vi "WildBugChilGru_V1.01.vi"() -> ()   [LabVIEW 2014]
uses:
  <vilib>/Utility/miscctls.llb/LVPointTypeDef.ctl
  <vilib>/Analysis/NI_AALBase.lvlib
  <vilib>/gmath/NI_Gmath.lvlib
  <vilib>/Analysis/NI_AALPro.lvlib
  <vilib>/Utility/xml.llb/Read From XML File(string).vi
  <vilib>/Utility/xml.llb/Write to XML File(string).vi
  <vilib>/Instr/_visa.llb/VISA Configure Serial Port (Instr).vi
  <vilib>/Analysis/3filter.llb/IIR Filter (DBL).vi
panel:
  in  "Registerkarte":T1(tab)
  in  "Zündung [Imp/U]":u8=1
  in  "Übersetzung ermitteln aus":T2(ring)
  in  "Getriebe [1:]":dbl=5.343
  in  "Reifenumfang [m]":dbl=1.222
  in  "Dauer [s]":dbl=5.0
  in  "nKuWe/nRolle":dbl=10.0
  in  "Lufttemperatur [°C]":dbl=20.0
  in  "Luftfeuchtigkeit [%]":dbl=50.0
  in  "Luftdruck [mbar]":dbl=1013.0
  in  "Messung Klimadaten":bool=TRUE
  in  "Gleitender Mittelwert":u8=35
  in  "Differenzenquotient":u8=12
  in  "Polynom":u8=15
  in  "n vom Gas [1/min]":dbl=5000.0
  in  "Rollengeber [Inkr/U]":u16=200
  in  "Rollenumfang [m]":dbl=0.613
  in  "Rollenträgheit [kgm²]":dbl=0.402
  in  "Recalc":bool
  in  "Ende":bool
  out "Datenspeicher":T3={"Fahrzeugdaten"="", "date/time string"="", "Rolle [Inkr/U]"=0, "Rollenumfang [m]"=0.0, "Rollenträgheit [kgm²]"=0.0, "Zündung [Imp/U]"=0, "Getriebe [1:]"=0.0, "Reifenumfang [m] "=0.0, "element"=0.0, "Gl. Mittelwert"=0, "Differenzenquotient"=0, "Polynom"=0, "element"=0.0, "element"=0.0, "Lufttemperatur [°C]"=0.0, "Luftfeuchtigkeit [%]"=0.0, "Luftdruck [mbar]"=0.0, [], [], "Best Polynomial Fit"=[], [], "Übersetzung ermitteln aus"=0, "[s]"=0.0, "nmin [1/min]"=0.0, "nmax [1/min]"=0.0, "n vom Gas [1/min]"=0.0, [], [], "Boolesch"=FALSE, "Serielle Schnittstelle"="COM4"}
  out "COM-Fehlerrate":string="0 / 0,0%"
  in  "Konfiguration:":bool
  in  "Speichern":bool
  in  "Drucken":bool
  out "Pmax":string="0,0 PS"
  out "Ergebnis":string="0,0 PS bei 0 1/min   |   0,0 Nm bei 0 1/min   |   vmax: 2147483647 km/h\nDIN 70020 k =1,000 (20 °C, 50 %, 1013 mbar)\n20.11.2016 20:05 "
  in  "Fahrzeugdaten":string="Hier die Fahrzeugdaten eingeben"
  out "XY-Graph":cluster{dbl[], dbl[]}[](graph)
  out "Untersetzung\nermittelt":bool
  out "Untersetzung":dbl format="%#.2f"
  in  "Start":bool
  out "Füllstand Lesepuffer":u64(slide) scale=1.0..100.0
  out "Hinterrad\n[km/h]":dbl(knob) scale=0.0..150.0
  out "Welle\n[1/min]":cluster{dbl, dbl}(knob) scale=0.0..12000.0
  out "Lesepuffer":string="\n"
  in  "Serielle Schnittstelle":refnum<visa-resource-name>="COM4"
  out "Untersetzung-Graph":dbl(graph)=2.6802446808510636 caption="Untersetzung"
  # "1. n konstant halten\n2. START\n3. n weiter halten\n4. bei GO: Vollgas\n5. vom Gas gehen"
  # "Zündung\nRolle"
  # "Untersetzung aus:"
  # "Eingabe <> Messen"
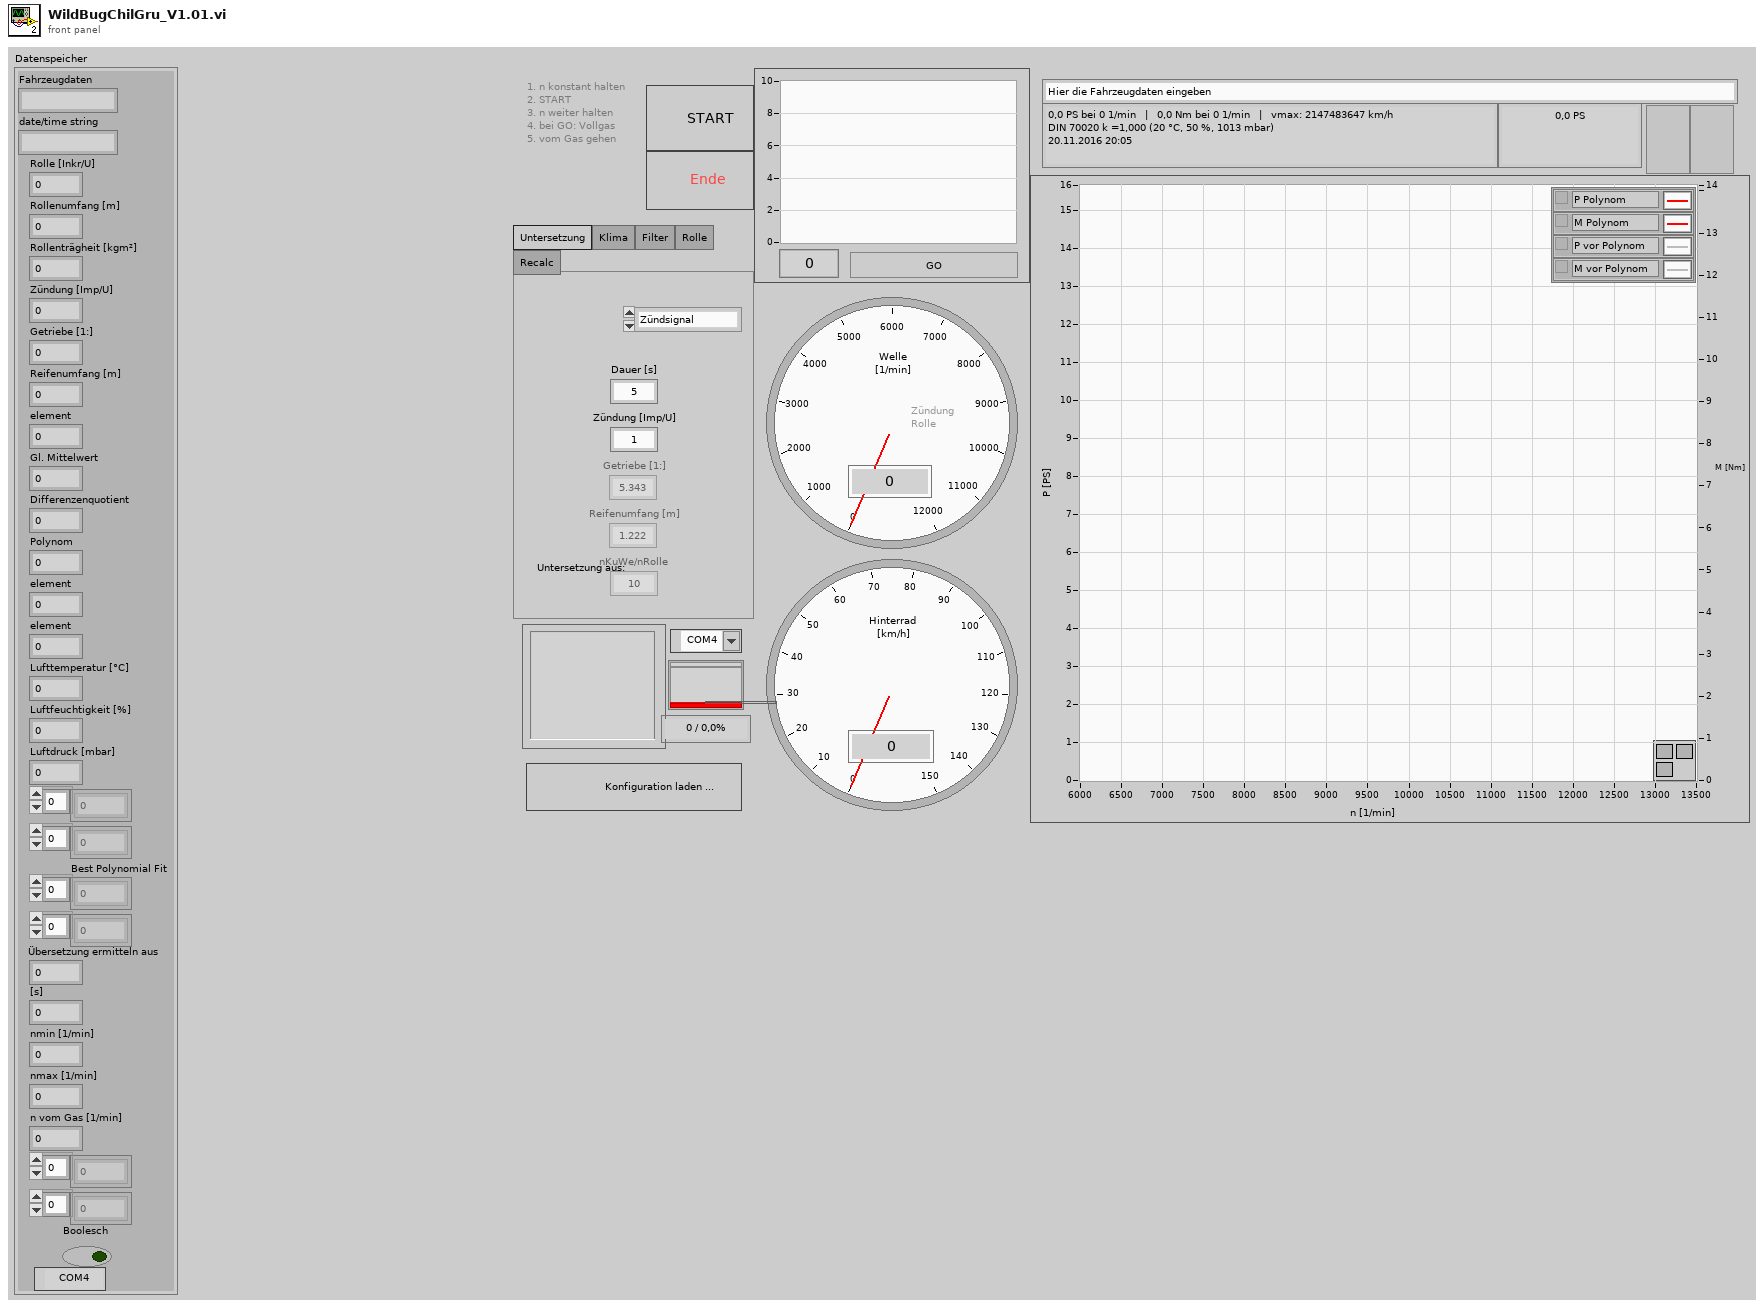
[diagram p1: front panel]
types:
  T1 = enum32{"Untersetzung", "Klima", "Filter", "Rolle", "Recalc"}
  T2 = enum8{"Zündsignal", "Getriebe & Reifen", "nKuWe / nRolle"}
  T3 = cluster{"Fahrzeugdaten":string, "date/time string":string, "Rolle [Inkr/U]":u16, "Rollenumfang [m]":dbl, "Rollenträgheit [kgm²]":dbl, "Zündung [Imp/U]":u8, "Getriebe [1:]":dbl, "Reifenumfang [m] ":dbl, "element":dbl, "Gl. Mittelwert":u8, "Differenzenquotient":u8, "Polynom":u8, "element":dbl, "element":dbl, "Lufttemperatur [°C]":dbl, "Luftfeuchtigkeit [%]":dbl, "Luftdruck [mbar]":dbl, dbl[], dbl[], "Best Polynomial Fit":dbl[], dbl[], "Übersetzung ermitteln aus":u8, "[s]":dbl, "nmin [1/min]":dbl, "nmax [1/min]":dbl, "n vom Gas [1/min]":dbl, dbl[], i32[], "Boolesch":bool, "Serielle Schnittstelle":refnum<visa-resource-name>}
  T4 = enum16{"Kleinste Quadrate", "Kleinestes absolutes Reiduum", "Biquadrat"}
  T5 = enum8{"Enabled", "Disabled", "Disabled and Grayed Out"}
  T6 = cluster{"Fahrzeugdaten":string, "date/time string":string, "Rollengeber [Inkr/U]":u16, "Rollenumfang [m]":dbl, "Rollenträgheit [kgm²]":dbl, "Zündung [Imp/U]":u8, "Getriebe [1:]":dbl, "Reifenumfang [m] ":dbl, "mean value":dbl, "Gleitender Mittelwert":u8, "Differenzenquotient":u8, "Polynom":u8, dbl, "element":dbl, "Lufttemperatur [°C]":dbl, "Luftfeuchtigkeit [%]":dbl, "Luftdruck [mbar]":dbl, dbl[], dbl[], "Best Polynomial Fit":dbl[], dbl[], "Übersetzung ermitteln aus":enum8{"Zündsignal", "Getriebe & Reifen", "nKuWe / nRolle"}, "Dauer [s]":dbl, dbl, dbl, "n vom Gas [1/min]":dbl, dbl[], i32[], "Messung Klimadaten":bool, "VISA resource name out":refnum<visa-resource-name>}
  T7 = typedef "LVPointTypeDef.ctl" = cluster{"Horizontal":i16, "Vertical":i16}
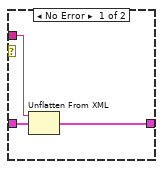
[diagram p2: hidden frame]
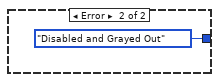
[diagram p3: hidden frame]
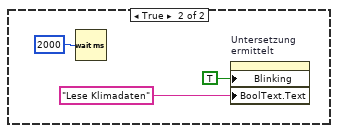
[diagram p5: hidden frame]
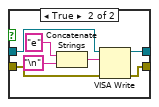
[diagram p6: hidden frame]
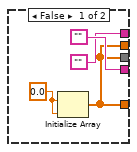
[diagram p8: hidden frame]
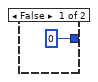
[diagram p9: hidden frame]
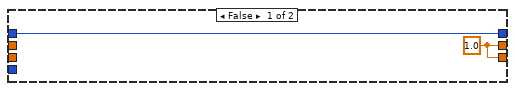
[diagram p11: hidden frame]
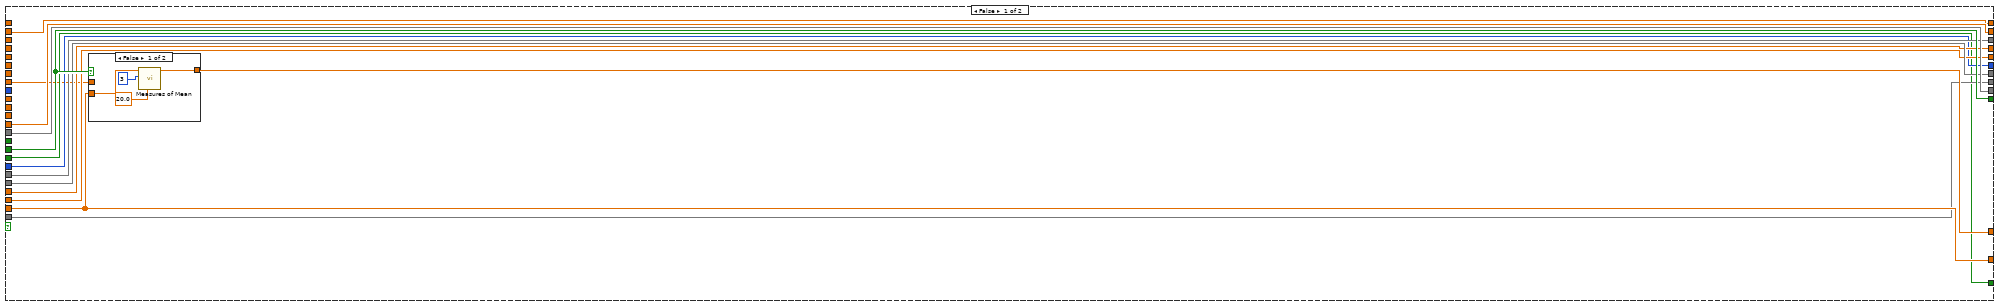
[diagram p12: hidden frame]
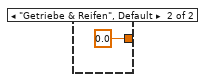
[diagram p16: hidden frame]
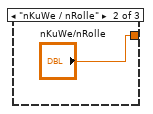
[diagram p18: hidden frame]
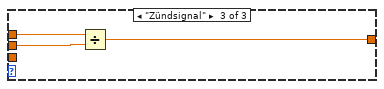
[diagram p19: hidden frame]
diagram:
  n1 = while {
    stop <- w1 stop-if-true
    n2 = event shown="[0] \"Start\": Wertänderung" {
      selector: _ -> [_ _]
      dyn-events: _ -> [_ _]
      timeout: _ -> [_ _]
      tunnel: [_ TRUE] -> w1
      event "Start": Value Change {
        n3 = event-data() -> ("NewVal"=w2:bool)  [unwired: 1 in, 5 out]
        n4 = case shown="True" w2 {
          frame False {
          }
          frame True {
            n5 = flat-sequence {
              tunnel: [w133] -> w118
              tunnel: [w132] -> w117
              tunnel: ["Messung Klimadaten"] -> w116
              tunnel: w118 -> [w146]
              tunnel: w117 -> [w145]
              tunnel: [0] -> w115
              tunnel: [1.0 ("element")] -> w114
              tunnel: [w143] -> w113
              tunnel: [w157] -> w112
              tunnel: [0] -> w111
              tunnel: [w143] -> w110
              tunnel: [-5] -> w109
              tunnel: [w154] -> w108
              tunnel: [w152] -> w107
              tunnel: [w151] -> w106
              tunnel: [0.0] -> w105
              tunnel: [w146] -> w104
              tunnel: [w145] -> w103
              tunnel: w116 -> [w144]
              tunnel: [w144] -> w102
              tunnel: w115 -> [w183]
              tunnel: [w183] -> w101
              tunnel: w114 -> [w182]
              tunnel: [w182] -> w100
              tunnel: w113 -> [w181]
              tunnel: [w181] -> w99
              tunnel: w112 -> [w180]
              tunnel: [w180] -> w98
              tunnel: w111 -> [w179]
              tunnel: [w179] -> w97
              tunnel: w110 -> [w178]
              tunnel: [w178] -> w96
              tunnel: w109 -> [w177]
              tunnel: [w177] -> w95
              tunnel: w108 -> [w176]
              tunnel: [w176] -> w94
              tunnel: w107 -> [w175]
              tunnel: [w175] -> w93
              tunnel: w106 -> [w174]
              tunnel: [w174] -> w92
              tunnel: w105 -> [w173]
              tunnel: [w173] -> w91
              tunnel: w104 -> [w172]
              tunnel: [w169] -> w90
              tunnel: w103 -> [w171]
              tunnel: [w170] -> w89
              tunnel: [w168] -> w88
              tunnel: w102 -> [w168]
              tunnel: w101 -> [w207]
              tunnel: [w207] -> w87
              tunnel: w100 -> [w206]
              tunnel: [w206] -> w86
              tunnel: w99 -> [w205]
              tunnel: [w205] -> w85
              tunnel: w98 -> [w204]
              tunnel: [w204] -> w84
              tunnel: w97 -> [w203]
              tunnel: [w203] -> w83
              tunnel: w96 -> [w202]
              tunnel: [w202] -> w82
              tunnel: w95 -> [w201]
              tunnel: [w201] -> w81
              tunnel: w94 -> [w200]
              tunnel: [w200] -> w80
              tunnel: w93 -> [w199]
              tunnel: [w199] -> w79
              tunnel: w92 -> [w198]
              tunnel: [w198] -> w78
              tunnel: w91 -> [w197]
              tunnel: [w197] -> w77
              tunnel: w90 -> [w196]
              tunnel: [w196] -> w76
              tunnel: w89 -> [w195]
              tunnel: [w195] -> w75
              tunnel: w88 -> [w193]
              tunnel: [w193] -> w74
              tunnel: w87 -> [w223]
              tunnel: [w223] -> w73
              tunnel: w86 -> [w222]
              tunnel: [w222] -> w72
              tunnel: w85 -> [w221]
              tunnel: [w221] -> w71
              tunnel: w84 -> [w220]
              tunnel: [w220] -> w70
              tunnel: w83 -> [w219]
              tunnel: [w219] -> w69
              tunnel: w82 -> [w218]
              tunnel: [w218] -> w68
              tunnel: w81 -> [w217]
              tunnel: [w217] -> w67
              tunnel: w80 -> [w216]
              tunnel: [w216] -> w66
              tunnel: w79 -> [w215]
              tunnel: [w215] -> w65
              tunnel: w78 -> [w214]
              tunnel: [w214] -> w64
              tunnel: w77 -> [w213]
              tunnel: [w213] -> w63
              tunnel: w76 -> [w212]
              tunnel: [w211] -> w62
              tunnel: w75 -> [w209]
              tunnel: [w210] -> w61
              tunnel: w74 -> [w208]
              tunnel: w73 -> [w297]
              tunnel: w72 -> [w296]
              tunnel: w71 -> [w295]
              tunnel: w70 -> [w294]
              tunnel: w69 -> [w293]
              tunnel: w68 -> [w292]
              tunnel: w67 -> [w291]
              tunnel: w66 -> [w290]
              tunnel: w65 -> [w289]
              tunnel: w64 -> [w288]
              tunnel: w63 -> [w287]
              tunnel: w62 -> [w252]
              tunnel: [w297] -> w60
              tunnel: [w296] -> w59
              tunnel: [w295] -> w58
              tunnel: [w294] -> w57
              tunnel: [w293] -> w56
              tunnel: [w292] -> w55
              tunnel: [w291] -> w54
              tunnel: [w290] -> w53
              tunnel: [w289] -> w52
              tunnel: [w288] -> w51
              tunnel: [w287] -> w50
              tunnel: [w252] -> w49
              tunnel: [w251] -> w48
              tunnel: [w286] -> w47
              tunnel: [w285] -> w46
              tunnel: [w284] -> w45
              tunnel: ["Gleitender Mittelwert"] -> w44
              tunnel: w61 -> [w251]
              tunnel: [w306] -> w10
              tunnel: [w307] -> w11
              tunnel: [w308] -> w12
              tunnel: [w309] -> w13
              tunnel: [w300] -> w8
              tunnel: [w299] -> w9
              tunnel: [w310] -> w14
              tunnel: [w311] -> w15
              tunnel: [w312] -> w17
              tunnel: [w313] -> w19
              tunnel: [w314] -> w20
              tunnel: [w315] -> w21
              tunnel: [w316] -> w38
              tunnel: [w317] -> w40
              tunnel: [w318] -> w41
              tunnel: [w319] -> w42
              tunnel: [w320] -> w43
              tunnel: w60 -> [w320]
              tunnel: w59 -> [w319]
              tunnel: w58 -> [w318]
              tunnel: w57 -> [w317]
              tunnel: w56 -> [w316]
              tunnel: w55 -> [w315]
              tunnel: w54 -> [w314]
              tunnel: w53 -> [w313]
              tunnel: w52 -> [w312]
              tunnel: w51 -> [w311]
              tunnel: w50 -> [w310]
              tunnel: w49 -> [w302]
              tunnel: w48 -> [w301]
              tunnel: w47 -> [w309]
              tunnel: w46 -> [w308]
              tunnel: w45 -> [w307]
              tunnel: w44 -> [w306]
              frame #0 {
                w138 = u16 0 items=["None", "XON/XOFF", "RTS/CTS", "XON/XOFF & RTS/CTS", "DTR/DSR", "XON/XOFF & DTR/DSR"] ("flow control (0:none)")
                w139 = u16 10 items=["1.0"=10, "1.5"=15, "2.0"=20] ("stop bits (10: 1 bit)")
                w131 = FALSE  # Enable Termination Char (T)
                w134 = u32 10000  # timeout (10sec)
                n6 = call-poly "VISA Configure Serial Port"("VISA resource name"="Serielle Schnittstelle", "timeout (10sec)"=w134, "Enable Termination\nChar (T)"=w131, "baud rate (9600)"=u32 115200 ("baudrate (250000)"), "data bits (8)"=u16 8, "parity (0:none)"=enum16{"None", "Odd", "Even", "Mark", "Space"}."None", "stop bits (10: 1 bit)"=w139, "flow control (0:none)"=w138) -> ("VISA resource name out"=w136:refnum<visa-resource-name>, "error out"=w135:errorcluster)  [unwired: 6 in]
                n7 = VISA Clear(VISA resource name=w136, error in (no error)=w135) -> (VISA resource name out=w133:refnum<visa-resource-name>, error out=w132:errorcluster)
              }
              frame #1 {
                w147 = T5."Disabled and Grayed Out" ("Deaktiviert")
                w150 = 0.0  # Graphen löschen
                w153 = 0
                w158 = 0.0
                w143 = FALSE
                w151 = ""
                n8 = case shown="False" w144 {
                  frame False {
                    n9 = property on="Untersetzung\nermittelt" class="Bool. (strikt)"("Blinking"=TRUE ("Blinkend"), "BoolText.Text"="Initialisiere" ("Beschriftung.Text")) -> ()  [unwired: 2 in, 2 out]
                  }
                  frame True {
                    n10 = Wait (ms)(milliseconds to wait=u32 2000 ("Zu wartende ms")) -> ()  [unwired: 1 out]
                    n11 = property on="Untersetzung\nermittelt" class="Bool. (strikt)"("Blinking"=TRUE ("Blinkend"), "BoolText.Text"="Lese Klimadaten" ("Beschriftung.Text")) -> ()  [unwired: 2 in, 2 out]
                  }
                }
                n12 = Build Array(w150) -> (w149:dbl[])
                n13 = property on="Untersetzung-Graph" class="SVDiagr (strikt)"("History Data"=w149) -> ()  [unwired: 2 in, 2 out]
                n14 = property on="Drucken" class="Bool. (strikt)"("DisabledEnum"=w147) -> ()  [unwired: 2 in, 2 out]
                n15 = property on="Übersetzung ermitteln aus" class="Enum (strikt)"("DisabledEnum"=w147) -> ()  [unwired: 2 in, 2 out]
                n16 = property on="Konfiguration:" class="Bool. (strikt)"("DisabledEnum"=w147) -> ()  [unwired: 2 in, 2 out]
                n17 = property on="Ende" class="Bool. (strikt)"("DisabledEnum"=w147) -> ()  [unwired: 2 in, 2 out]
                n18 = property on="Speichern" class="Bool. (strikt)"("DisabledEnum"=w147) -> ()  [unwired: 2 in, 2 out]
                n19 = local write "Pmax"(w151) -> ()
                n20 = local write "COM-Fehlerrate"(w151) -> ()
                n21 = local write "Ergebnis"(w151) -> ()
                n22 = Initialize Array(w158, w158) -> (w157:dbl[])
                n23 = Initialize Array(0.0 ("y"), 0) -> (w154:dbl[])
                n24 = Initialize Array(w153, w153) -> (w152:i32[])
              }
              frame #2 {
                n25 = case shown="False" w168 {
                  tunnel: w172 -> [w185 w189]
                  tunnel: w171 -> [w184 w188]
                  tunnel: [w184 w187] -> w170
                  tunnel: [w185 w186] -> w169
                  frame False {
                  }
                  frame True {
                    n26 = Concatenate Strings("e" ("String"), "\n") -> (w192:string)
                    n27 = VISA Write(VISA resource name=w189, write buffer=w192, error in (no error)=w188) -> (VISA resource name out=w186:refnum<visa-resource-name>, error out=w187:errorcluster)  [unwired: 1 out]
                  }
                }
              }
              frame #3 {
                n28 = Wait (ms)(milliseconds to wait=u32 500 ("Zu wartende ms")) -> ()  [unwired: 1 out]
              }
              frame #4 {
                n29 = case shown="True" w208 {
                  tunnel: w212 -> [w225 w246]
                  tunnel: [w225 w245] -> w211
                  tunnel: [w224 w244] -> w210
                  tunnel: w209 -> [w224 w243]
                  frame False {
                  }
                  frame True {
                    w228 = ";" ("Regulärer Ausdruck")
                    n30 = property class="Instr"(reference=w246, error in=w243) -> (reference out=w249:refnum<visa-resource-name>, error out=w248:errorcluster, "Serial Settings:Number of Bytes at Serial Port"=w247:u32)
                    n31 = VISA Read(VISA resource name=w249, byte count=w247, error in (no error)=w248) -> (VISA resource name out=w245:refnum<visa-resource-name>, read buffer=w240:string, error out=w244:errorcluster)  [unwired: 1 out]
                    n32 = Search and Replace String(replace all?=TRUE ("Alle ersetzen? (F)"), input string=w240, search string="." ("Such-String"), replace string="," ("Ersetzungs-String (\"\")")) -> (result string=w233:string)  [unwired: 4 in, 3 out]
                    n33 = Match Pattern(string=w233, regular expression=w228) -> (before substring=w231:string, after substring=w232:string)  [unwired: 1 in, 2 out]
                    n34 = Match Pattern(string=w232, regular expression=w228) -> (before substring=w230:string, after substring=w229:string)  [unwired: 1 in, 2 out]
                    n35 = Fract/Exp String To Number(string=w231, offset=0 ("Offset")) -> (number=w239:dbl)  [unwired: 2 in, 1 out]
                    n36 = local write "Lufttemperatur [°C]"(w239) -> ()
                    n37 = Fract/Exp String To Number(string=w230) -> (number=w236:dbl)  [unwired: 3 in, 1 out]
                    n38 = Match Pattern(string=w229, regular expression=w228) -> (before substring=w227:string)  [unwired: 1 in, 3 out]
                    n39 = Fract/Exp String To Number(string=w227) -> (number=w238:dbl)  [unwired: 3 in, 1 out]
                    n40 = Divide(x=w236, y=100.0 ("x")) -> (x/y=w237:dbl)
                    n41 = local write "Luftdruck [mbar]"(w237) -> ()
                    n42 = local write "Luftfeuchtigkeit [%]"(w238) -> ()
                  }
                }
              }
              frame #5 {
                n43 = Wait (ms)(milliseconds to wait=u32 2000 ("Zu wartende ms")) -> ()  [unwired: 1 out]
                n44 = Add(x="Lufttemperatur [°C]", y=273.15) -> (x+y=w267:dbl)
                n45 = Divide ("M_Welle [Nm]")(x=300.0, y=w267) -> (x/y=w270:dbl)
                n46 = Multiply(x="Luftfeuchtigkeit [%]", y=0.01) -> (x*y=w281:dbl)
                n47 = Divide ("M_Welle [Nm]")(x=w267, y=293.15) -> (x/y=w265:dbl)
                n48 = Multiply(x=w281, y=240800000000.0) -> (x*y=w255:dbl)
                n49 = Power Of X(1:w270, 2:5.0) -> (0:w268:dbl)
                n50 = Multiply(x=w255, y=w268) -> (x*y=w275:dbl)
                n51 = Multiply(x=w270, y=-22.644) -> (x*y=w276:dbl)
                n52 = Power Of X(1:w265, 2:0.5) -> (0:w262:dbl)
                n53 = Exponential(1:w276) -> (0:w274:dbl)
                n54 = Multiply(x=w275, y=w274) -> (x*y=w273:dbl)
                n55 = Subtract "p_Trocken [mbar]"(x="Luftdruck [mbar]", y=w273) -> (x-y=w271:dbl)
                n56 = Divide ("M_Welle [Nm]")(x=1013.0, y=w271) -> (x/y=w263:dbl)
                n57 = Multiply "Korrekturfaktor DIN 70020"(x=w263, y=w262) -> (x*y=w286:dbl)
                n58 = Divide(x="Gleitender Mittelwert", y=2) -> (x/y=w259:dbl)
                n59 = Round Toward -Infinity(1:w259) -> (0:w258:dbl)
                n60 = call <vilib>:"Smoothing Filter Coefficients.vi"("shape"=1, "half-width"=w258, "type"=0) -> ("forward coefficients"=w284:dbl[], "reverse coefficients"=w285:dbl[])  [unwired: 6 in, 1 out]
              }
              frame #6 {
                n61 = Concatenate Strings("m" ("String"), "\n") -> (w305:string)
                n62 = property on="Untersetzung\nermittelt" class="Bool. (strikt)"("Blinking"=FALSE ("Blinkend")) -> ()  [unwired: 2 in, 2 out]
                n63 = VISA Write(VISA resource name=w302, write buffer=w305, error in (no error)=w301) -> (VISA resource name out=w299:refnum<visa-resource-name>, error out=w300:errorcluster)  [unwired: 1 out]
              }
            }
            n64 = while {
              tunnel: w9 -> [w453]
              tunnel: w8 -> [w452]
              shift-right: [w523] -> _
              shift-left: w15 -> [w468]
              shift-right: [w518] -> _
              shift-left: w14 -> [w522]
              shift-right: [w517] -> _
              shift-left: w14 -> [w521]
              shift-right: [w472] -> _
              shift-left: w14 -> [w520]
              shift-right: [w499] -> _
              shift-left: w43 -> [w519]
              shift-right: [w460] -> w26
              shift-left: w42 -> [_]
              shift-right: [w478] -> w30
              shift-left: w14 -> [w500]
              shift-right: [w510] -> w28
              shift-left: w14 -> [w474]
              shift-right: [w473] -> _
              shift-left: w19 -> [w514]
              shift-right: [w511] -> _
              shift-left: w41 -> [w488]
              shift-right: [w454] -> _
              shift-left: w40 -> [_]
              shift-right: [w459] -> _
              shift-left: w40 -> [_]
              shift-right: [w509] -> w29
              shift-left: w40 -> [w507]
              shift-right: [w508] -> _
              shift-left: w40 -> [w506]
              shift-right: [w494] -> w37
              shift-left: w19 -> [w505]
              shift-right: [w498] -> _
              shift-left: w19 -> [w503]
              shift-right: [w497] -> w33
              shift-left: w19 -> [w504]
              shift-right: [w496] -> w36
              shift-left: w19 -> [w502]
              shift-right: [w495] -> w35
              shift-left: w19 -> [w501]
              tunnel: [w493] -> w39
              shift-right: [w489] -> w34
              shift-left: w38 -> [w491]
              tunnel: [w492] -> w5
              tunnel: ["n vom Gas [1/min]"] -> w32
              tunnel: ["Rollenumfang [m]"] -> w31
              tunnel: ["Rollenumfang [m]"] -> w25
              shift-right: [w485] -> _
              shift-left: w21 -> [w451]
              shift-right: [w479] -> _
              shift-left: w20 -> [w484]
              shift-right: [w480] -> _
              shift-left: w14 -> [w483]
              shift-right: [w481] -> _
              shift-left: w14 -> [w482]
              shift-right: [w477] -> w18
              shift-left: w19 -> [w476]
              shift-right: [w471] -> _
              shift-left: _ -> [w470]
              shift-right: [w475] -> w16
              shift-left: w17 -> [w469]
              tunnel: [w467] -> w6
              tunnel: w13 -> [w460]
              tunnel: w12 -> [w454]
              tunnel: w11 -> [w459]
              tunnel: w10 -> [w458]
              stop <- w493 stop-if-true
              n65 = property class="Instr"(reference=w453, error in=w452) -> (reference out=w463:refnum<visa-resource-name>, error out=w462:errorcluster, "Serial Settings:Number of Bytes at Serial Port"=w465:u32)
              n66 = Greater?(x=w465, y=u32 1 ("min. Bytes")) -> (0:w461:bool)
              n67 = case shown="True" w461 {
                tunnel: w465 -> [_ w525]
                tunnel: [u32 0 ("Bytes at Port") w525] -> w464
                frame False {
                }
                frame True {
                }
              }
              n68 = case shown="1.." w464 {
                selector: w464 -> [_ w778]
                tunnel: [w728 w772] -> w492
                tunnel: [w727 w773] -> w467
                tunnel: [w732 w774] -> w517
                tunnel: [w733 w771] -> w518
                tunnel: w468 -> [w734 w769]
                tunnel: [w734 w767] -> w523
                tunnel: w522 -> [w733 w759]
                tunnel: w521 -> [w732 w758]
                tunnel: [w729 w757] -> w472
                tunnel: w520 -> [w729 w756]
                tunnel: w519 -> [w731 _]
                tunnel: [w731 w739] -> w499
                tunnel: [w730 w745] -> w471
                tunnel: w470 -> [w730 w744]
                tunnel: w463 -> [w727 w736]
                tunnel: w462 -> [w728 w735]
                frame 0, Default {
                  # "No data in from serial port - Nothing to do."
                }
                frame 1.. {
                  # "Hz Drum"
                  n69 = VISA Read(VISA resource name=w736, byte count=w778, error in (no error)=w735) -> (VISA resource name out=w773:refnum<visa-resource-name>, read buffer=w770:string, error out=w772:errorcluster)  [unwired: 1 out]
                  n70 = Concatenate Strings(w769, w770) -> (w741:string)
                  "Lesepuffer" <- w741
                  n71 = Spreadsheet String To Array(delimiter (Tab)="\n" ("regular expression"), format string="%s" ("regular expression"), spreadsheet string=w741, array type (2D Dbl)=string[] [] ("Array 2")) -> (array=w750:string[])
                  n72 = Match Pattern(string=w741, regular expression="[\\n]") -> (before substring=w748:string, after substring=w768:string, offset past match=w782:i32)  [unwired: 1 in, 1 out]
                  n73 = Array Size(array=w750) -> (size(s)=w754:i32)
                  n74 = Match Pattern(string=w748, regular expression="[;]") -> (before substring=w746:string, after substring=w747:string, offset past match=w743:i32)  [unwired: 1 in, 1 out]
                  n75 = Subtract "aktuelle Zeilenanzahl"(x=w754, y=1) -> (x-y=w739:i32)
                  n76 = property on="Füllstand Lesepuffer" class="Schieber (strikt)"() -> ("Scale.Maximum"=w738:dbl)  [unwired: 2 in, 2 out]
                  n77 = Match Pattern(string=w747, regular expression="[;]") -> (before substring=w777:string, after substring=w780:string, offset past match=w765:i32)  [unwired: 1 in, 1 out]
                  n78 = Match Pattern(string=w780, regular expression="[;]") -> (before substring=w776:string, after substring=w775:string, offset past match=w763:i32)  [unwired: 1 in, 1 out]
                  n79 = Greater Or Equal To 0?(x=w743) -> (x >= 0?=w742:bool)
                  n80 = Greater?(x=w739, y=w738) -> (0:w740:bool)
                  n81 = Greater Or Equal To 0?(x=w763) -> (x >= 0?=w762:bool)
                  n82 = Greater Or Equal To 0?(x=w765) -> (x >= 0?=w764:bool)
                  n83 = Greater Or Equal To 0?(x=w782) -> (x >= 0?=w766:bool)
                  n84 = Select(t=w739, s=w740, f=w738) -> (s? t:f=w737:dbl)
                  n85 = Build Array(w766, w764, w742, w762) -> (w761:bool[])
                  n86 = property on="Füllstand Lesepuffer" class="Schieber (strikt)"("Scale.Maximum"=w737) -> ()  [unwired: 2 in, 2 out]
                  n87 = And Array Elements(Boolean array=w761) -> (logical AND=w760:bool)
                  n88 = case shown="True" w760 {
                    tunnel: w777 -> [_ w793]
                    tunnel: w776 -> [_ w798]
                    tunnel: w775 -> [_ w797]
                    tunnel: [w786 w796] -> w774
                    tunnel: [w787 w795] -> w771
                    tunnel: w768 -> [_ w794]
                    tunnel: [w788 w794] -> w767
                    tunnel: w741 -> [w788 _]
                    tunnel: w759 -> [w787 _]
                    tunnel: w758 -> [w786 _]
                    tunnel: [w785 w792] -> w757
                    tunnel: w756 -> [w785 _]
                    tunnel: w746 -> [_ w791]
                    tunnel: [w784 w789] -> w745
                    tunnel: w744 -> [w784 _]
                    frame False {
                    }
                    frame True {
                      # "Cyclecounter"
                      # "Hz ComLevel"
                      # "ComLevel\nLevel 10 =   6Hz \nLevel 5 =   12Hz \nLevel 4 =   15Hz\nLevel 3 =   20Hz\nLevel 2 =   33Hz\nLevel 1 =   62Hz"
                      # "Hz Drum"
                      # "Hz Engine"
                      # "t4m"
                      n89 = Fract/Exp String To Number(string=w791) -> (number=w790:dbl)  [unwired: 3 in, 1 out]
                      n90 = Fract/Exp String To Number(string=w797) -> (number=w796:dbl)  [unwired: 3 in, 1 out]
                      n91 = Fract/Exp String To Number(string=w793) -> (number=w792:dbl)  [unwired: 3 in, 1 out]
                      n92 = To Long Integer(number=w790) -> (32bit integer=w789:i32)
                      n93 = Fract/Exp String To Number(string=w798) -> (number=w795:dbl)  [unwired: 3 in, 1 out]
                    }
                  }
                }
              }
              "Füllstand Lesepuffer" <- w499
              n94 = Not Equal?(x=w470, y=w471) -> (x != y?=w455:bool)
              n95 = case shown="True" w455 {
                tunnel: w484 -> [w529 w540]
                tunnel: [w529 w552] -> w479
                tunnel: w483 -> [w528 w551]
                tunnel: [w528 w537] -> w480
                tunnel: w482 -> [w527 w550]
                tunnel: [w527 w538] -> w481
                tunnel: w471 -> [_ w536]
                tunnel: w469 -> [w526 w535]
                tunnel: [w526 w539] -> w475
                frame False {
                }
                frame True {
                  n96 = Build Array (concatenate)(w535, w536) -> (w539:i32[])
                  n97 = Greater Or Equal To 0?(x=w540) -> (x >= 0?=w541:bool)
                  n98 = case shown="True" w541 {
                    tunnel: [w553 w564] -> w537
                    tunnel: [w553 w565] -> w538
                    tunnel: [w554 w556] -> w552
                    tunnel: w551 -> [_ w558]
                    tunnel: w550 -> [_ w566]
                    tunnel: w536 -> [w554 w555]
                    tunnel: w540 -> [_ w556]
                    frame False {
                      w553 = 1.0
                    }
                    frame True {
                      w562 = 65536.0
                      n99 = Add(x=w556, y=w558) -> (x+y=w557:dbl)
                      n100 = Increment(x=w566) -> (x+1=w565:dbl)
                      n101 = Divide(x=w557, y=w562) -> (x/y=w567:dbl)
                      n102 = Round Toward -Infinity(1:w567) -> (0:w563:dbl)
                      n103 = Multiply(x=w563, y=w562) -> (x*y=w561:dbl)
                      n104 = Add(x=w561, y=w555) -> (x+y=w560:dbl)
                      n105 = Increment(x=w560) -> (x+1=w559:dbl)
                      n106 = Subtract(x=w559, y=w556) -> (x-y=w564:dbl)
                    }
                  }
                  n107 = Subtract(x=w537, y=w538) -> (x-y=w532:dbl)
                  n108 = Decrement(x=w532) -> (x-1=w531:dbl)
                  n109 = Max & Min(x=0, y=w531) -> (max(x,y)=w530:dbl)  [unwired: 1 out]
                  n110 = Divide(x=w530, y=w537) -> (x/y=w544:dbl)
                  n111 = Greater Than 0?(x=w530) -> (x > 0?=w534:bool)
                  n112 = Select(t=u32 16711680, s=w534, f=u32 0) -> (s? t:f=w545:u32)
                  n113 = Multiply(x=w544, y=100.0) -> (x*y=w542:dbl)
                  n114 = Format Into String(format string="%d / %.1f%%" ("Format-String"), w530, w542) -> (resulting string=→"COM-Fehlerrate":string)  [unwired: 2 in, 1 out]
                  n115 = property on="COM-Fehlerrate" class="Str"("Text.TextColor"=w545) -> ()  [unwired: 2 in, 2 out]
                }
              }
              n116 = case "Case-Struktur" shown="True" w455 {
                tunnel: w518 -> [w708 w719]
                tunnel: w517 -> [w707 w718]
                tunnel: [w708 w717] -> w516
                tunnel: [w707 w716] -> w515
                tunnel: w472 -> [_ w710]
                tunnel: w500 -> [w706 _]
                tunnel: [w706 w709] -> w478
                tunnel: w474 -> [_ w715]
                tunnel: "Rollenumfang [m]" -> [_ w714]
                frame False {
                }
                frame True {
                  w726 = 60.0 ("y")
                  n117 = Reciprocal "Abtastzeit [s]"(x=w710) -> (1/x=w709:dbl)
                  n118 = Divide "R [1/s]"(x=w718, y="Rollengeber [Inkr/U]") -> (x/y=w725:dbl)
                  n119 = Divide(x=w719, y="Zündung [Imp/U]") -> (x/y=w722:dbl)
                  n120 = Multiply "nZ gemessen [1/min]"(x=w722, y=w726) -> (x*y=w717:dbl)
                  n121 = Multiply "nR [1/min]"(x=w726, y=w725) -> (x*y=w716:dbl)
                  n122 = Multiply "nZ berechnet [1/min]"(x=w716, y=w715) -> (x*y=w724:dbl)
                  n123 = Multiply "[m/min]"(x=w716, y=w714) -> (x*y=w720:dbl)
                  n124 = Multiply "[km/h]"(x=w720, y=0.06) -> (x*y=→"Hinterrad\n[km/h]":dbl)
                  n125 = Bundle(w717, w724) -> (→"Welle\n[1/min]":cluster{dbl, dbl})  [unwired: 1 in]
                }
              }
              n126 = case shown="True" w455 {
                tunnel: w516 -> [_ w637]
                tunnel: w515 -> [_ w636]
                tunnel: "Rollenumfang [m]" -> [_ w640]
                tunnel: [w579 w606] -> w510
                tunnel: w474 -> [w568 w606]
                tunnel: w488 -> [w580 w644]
                tunnel: w514 -> [w581 w643]
                tunnel: [w580 w597] -> w511
                tunnel: [w581 w642] -> w473
                tunnel: w454 -> [_ w639]
                tunnel: w459 -> [_ w638]
                tunnel: [w578 w592] -> w509
                tunnel: [w577 w590] -> w508
                tunnel: w507 -> [w578 w635]
                tunnel: w506 -> [w577 _]
                tunnel: w458 -> [_ w588]
                tunnel: [w576 w612] -> w494
                tunnel: w505 -> [w576 _]
                tunnel: [w575 w627] -> w498
                tunnel: w503 -> [w575 _]
                tunnel: w500 -> [_ w625]
                tunnel: [w574 w613] -> w497
                tunnel: w504 -> [w574 _]
                tunnel: [w573 w629] -> w496
                tunnel: w502 -> [w573 _]
                tunnel: [w572 w628] -> w495
                tunnel: w501 -> [w572 _]
                tunnel: w460 -> [_ w617]
                tunnel: w491 -> [w571 w611]
                tunnel: "n vom Gas [1/min]" -> [_ w599]
                tunnel: [w571 w610] -> w489
                tunnel: w488 -> [_ w609]
                tunnel: w451 -> [w570 w605]
                tunnel: [w570 w604] -> w485
                tunnel: w478 -> [_ w603]
                tunnel: [w569 w602] -> w477
                tunnel: w476 -> [w569 w601]
                frame False {
                  n127 = case shown="False" w580 {
                    tunnel: w581 -> [w585 _]
                    tunnel: [w584 w586] -> w579
                    tunnel: w568 -> [_ w586]
                    frame False {
                      n128 = call <vilib>:"Measures of Mean.vi"("percent (trim)"=20.0, "type"=3, "x array"=w585) -> ("mean value"=w584:dbl)  [unwired: 7 in, 1 out]
                    }
                    frame True {
                    }
                  }
                }
                frame True {
                  w620 = 0.00135962  # [W] in [PS]
                  w631 = 0.10471975511965978  # 2*Pi/60
                  n129 = Build Array (concatenate) "akt. dT in Array einfügen"(w601, w603) -> (w602:dbl[])
                  n130 = Build Array (concatenate) "akt. Rollendrehzahl\nin Array einfügen"(w635, w636) -> (w592:dbl[])
                  n131 = local read "Übersetzung ermitteln aus"() -> (w587:T2)
                  n132 = Index Array(array=w592, index=1 ("Index")) -> (element=w595:dbl)
                  n133 = case shown="\"Getriebe & Reifen\"" w587 {
                    tunnel: w637 -> [_ _ w705]
                    tunnel: w636 -> [_ _ w704]
                    tunnel: [w700 "nKuWe/nRolle" w703] -> w641
                    tunnel: w640 -> [w701 _ _]
                    frame "Getriebe & Reifen" {
                      n134 = Divide(x=w701, y="Reifenumfang [m]") -> (x/y=w699:dbl)
                      n135 = Multiply(x=w699, y="Getriebe [1:]") -> (x*y=w700:dbl)
                    }
                    frame "nKuWe / nRolle" {
                    }
                    frame "Zündsignal" {
                      n136 = Divide(x=w705, y=w704) -> (x/y=w703:dbl)
                    }
                  }
                  n137 = Initialize Array(w595, w588) -> (w594:dbl[])
                  n138 = Insert Into Array(array=w592, index=0 ("Index"), new element=w594) -> (w591:dbl[])
                  n139 = call-poly <vilib>:"IIR Filter.vi"("Forward Coefficients"=w638, "Reverse Coefficients"=w639, "X"=w591) -> ("Filtered X"=w589:dbl[])  [unwired: 1 in, 1 out]
                  n140 = Array Subset(array=w589, index=w588) -> (w590:dbl[])  [unwired: 1 in]
                  n141 = Multiply(x=2.0, y=w625) -> (x*y=w624:dbl)
                  n142 = case shown="False" w644 {
                    selector: w644 -> [_ w696]
                    tunnel: w641 -> [w685 _]
                    tunnel: w643 -> [w687 w695]
                    tunnel: [w681 w696] -> w634
                    tunnel: [w686 w695] -> w642
                    tunnel: w605 -> [w684 w694]
                    tunnel: [w681 w694] -> w604
                    tunnel: w587 -> [w682 _]
                    frame False {
                      n143 = Build Array (concatenate)(w687, w685) -> (w686:dbl[])
                      n144 = case shown="\"Zündsignal\"" w682 {
                        tunnel: ["Dauer [s]" 0.0 ("Dauer [s]")] -> w683
                        frame "Zündsignal" {
                          n145 = property on="Untersetzung\nermittelt" class="Bool. (strikt)"("Blinking"=TRUE ("Blinkend"), "BoolText.Text"="Ermittle Übersetzung" ("Boolescher Text.Text")) -> ()  [unwired: 2 in, 2 out]
                        }
                        frame "Getriebe & Reifen", Default {
                        }
                      }
                      n146 = call "Verstrichene Zeit"("Time Target (s)"=w683, "Reset"=w684) -> ("Time has Elapsed"=w681:bool)  [unwired: 10 in, 7 out]
                      n147 = case shown="True" w681 {
                        frame False {
                        }
                        frame True {
                          n148 = property on="Untersetzung\nermittelt" class="Bool. (strikt)"("Blinking"=FALSE ("Blinkend"), "BoolText.Text"="Go" ("Boolescher Text.Text")) -> ()  [unwired: 2 in, 2 out]
                        }
                      }
                      "Untersetzung-Graph" <- w685
                    }
                    frame True {
                    }
                  }
                  n149 = Array Size "Array-Größe"(array=w590) -> (size(s)=w632:i32)
                  n150 = Square(x=w606) -> (x^2=w630:dbl)
                  n151 = Multiply(x=w590, y=w606) -> (x*y=w612:dbl[])
                  n152 = Multiply(x=w612, y=w631) -> (x*y=w627:dbl[])
                  n153 = Greater?(x=w632, y=w588) -> (0:w633:bool)
                  n154 = Divide(x="Rollenträgheit [kgm²]", y=w630) -> (x/y=w618:dbl)
                  n155 = Multiply(x=w618, y=w617) -> (x*y=w616:dbl)
                  n156 = And(x=w634, y=w633) -> (x .and. y?=w597:bool)
                  n157 = Array Size "Array-Größe"(array=w627) -> (size(s)=w615:i32)
                  n158 = Decrement(x=w615) -> (x-1=w614:i32)
                  n159 = Select(t=w599, s=w597, f=1000000.0) -> (s? t:f=w600:dbl)
                  n160 = Initialize Array(0.0 ("y"), 0) -> (w621:dbl[])
                  n161 = for {
                    N: w615 -> [_]
                    tunnel: "Differenzenquotient" -> [w656]
                    tunnel: w627 -> [w664]
                    tunnel: w614 -> [w655]
                    tunnel: w624 -> [w665]
                    shift-right: [w661] -> w613
                    shift-left: w621 -> [w662]
                    tunnel: w612 -> [w659] mode=indexing
                    tunnel: w611 -> [w647]
                    tunnel: w600 -> [w658]
                    tunnel: [w648] -> w610
                    tunnel: w609 -> [w645]
                    i -> [w649]
                    stop <- w646 stop-if-true
                    n162 = Subtract(x=w655, y=w656) -> (x-y=w657:i32)
                    n163 = Subtract(x=w649, y=w656) -> (x-y=w678:i32)
                    n164 = Add(x=w649, y=w656) -> (x+y=w672:i32)
                    n165 = Greater Or Equal?(x=w649, y=w656) -> (x >= y?=w652:bool)
                    n166 = Greater?(x=w659, y=w658) -> (0:w660:bool)
                    n167 = Max & Min(x=w655, y=w672) -> (min(x,y)=w673:i32)  [unwired: 1 out]
                    n168 = Max & Min(x=w678, y=0) -> (max(x,y)=w676:i32)  [unwired: 1 out]
                    n169 = Subtract(x=w673, y=w649) -> (x-y=w674:i32)
                    n170 = Less Or Equal?(x=w649, y=w657) -> (x <= y?=w653:bool)
                    n171 = Subtract(x=w649, y=w676) -> (x-y=w675:i32)
                    n172 = Max & Min(x=w675, y=w674) -> (min(x,y)=w666:i32)  [unwired: 1 out]
                    n173 = Add(x=w649, y=w666) -> (x+y=w671:i32)
                    n174 = Subtract(x=w649, y=w666) -> (x-y=w670:i32)
                    n175 = Multiply(x=w666, y=w665) -> (x*y=w663:dbl)
                    n176 = Index Array(array=w664, index=w671) -> (element=w668:dbl)
                    n177 = Index Array(array=w664, index=w670) -> (element=w669:dbl)
                    n178 = Subtract(x=w668, y=w669) -> (x-y=w667:dbl)
                    n179 = Divide(x=w667, y=w663) -> (x/y=w654:dbl)
                    n180 = Less Than 0?(x=w654) -> (x < 0?=w651:bool)
                    n181 = Less Or Equal To 0?(x=w647) -> (x <= 0?=w650:bool)
                    n182 = Build Array (concatenate)(w662, w654) -> (w661:dbl[])
                    n183 = Compound Arithmetic op=AND(w651, w660, w650, w652, w653, w645) -> (w646:bool)
                    n184 = case shown="True" w646 {
                      tunnel: w649 -> [_ w680]
                      tunnel: [w679 w680] -> w648
                      tunnel: w647 -> [w679 _]
                      frame False {
                      }
                      frame True {
                      }
                    }
                  }
                  n185 = Multiply(x=w613, y=w616) -> (x*y=w629:dbl[])
                  n186 = Multiply(x=w627, y=w629) -> (x*y=w619:dbl[])
                  n187 = Multiply(x=w620, y=w619) -> (x*y=w628:dbl[])
                }
              }
              "Untersetzung\nermittelt" <- w511
              n188 = local read "Start"() -> (w457:bool)
              n189 = Greater Than 0?(x=w489) -> (x > 0?=w490:bool)
              n190 = Not(x=w457) -> (.not. x?=w456:bool)
              n191 = Select(t=w510, s=w511, f=0.0) -> (s? t:f=→"Untersetzung":dbl)
              n192 = Or(x=w490, y=w456) -> (x .or. y?=w493:bool)
            }
            n193 = VISA Clear(VISA resource name=w6, error in (no error)=w5) -> (VISA resource name out=w3:refnum<visa-resource-name>, error out=w7:errorcluster)
            n194 = VISA Close(VISA resource name=w3, error in (no error)=w7) -> ()  [unwired: 1 out]
            n195 = case shown="True" w39 {
              tunnel: w37 -> [_ w427]
              tunnel: w36 -> [_ w432]
              tunnel: w35 -> [_ w431]
              tunnel: w34 -> [_ w403]
              tunnel: w33 -> [_ w428]
              tunnel: w32 -> [_ w426]
              tunnel: w31 -> [_ w420]
              tunnel: w26 -> [_ w406]
              tunnel: ["" w405] -> w27
              tunnel: w28 -> [_ w404]
              tunnel: ["" w402] -> _
              tunnel: [w366 w379] -> w24
              tunnel: [w366 w378] -> w23
              tunnel: [w366 w377] -> w22
              frame False {
                w367 = 0.0
                n196 = Initialize Array(w367, w367) -> (w366:dbl[])
              }
              frame True {
                w391 = 735.498  # PS in W
                w397 = 0.10471975511965978  # w = (2 * Pi / 60) * n
                w401 = 0
                n197 = Array Subset "P"(array=w431, length=w403) -> (w423:dbl[])  [unwired: 1 in]
                n198 = Array Subset "M"(array=w432, length=w403) -> (w424:dbl[])  [unwired: 1 in]
                n199 = Array Subset "alpha"(array=w428, length=w403) -> (w429:dbl[])  [unwired: 1 in]
                n200 = Array Subset "n"(array=w427, length=w403) -> (w425:dbl[])  [unwired: 1 in]
                n201 = property on="Pmax" class="Str"("Text.FontSize"=48) -> ()  [unwired: 2 in, 2 out]
                n202 = property on="Ergebnis" class="Str"("Text.FontSize"=18) -> ()  [unwired: 2 in, 2 out]
                n203 = Array Size(array=w429) -> (size(s)=w430:i32)
                n204 = for {
                  N: w430 -> [w450]
                  tunnel: w428 -> [w447]
                  tunnel: w427 -> [w444]
                  tunnel: w426 -> [w441]
                  tunnel: [w439] -> w399
                  i -> [w445]
                  stop <- w440 stop-if-true
                  n205 = Decrement(x=w450) -> (x-1=w449:i32)
                  n206 = Subtract(x=w449, y=w445) -> (x-y=w439:i32)
                  n207 = Index Array(array=w447, index=w439) -> (element=w448:dbl)
                  n208 = Index Array(array=w444, index=w439) -> (element=w443:dbl)
                  n209 = Less?(x=w443, y=w441) -> (x < y?=w442:bool)
                  n210 = Less Or Equal To 0?(x=w448) -> (x <= 0?=w446:bool)
                  n211 = And(x=w446, y=w442) -> (x .and. y?=w440:bool)
                }
                n212 = Increment(x=w399) -> (x+1=w398:i32)
                n213 = Array Subset "P"(array=w423, index=w398) -> (w400:dbl[])  [unwired: 1 in]
                n214 = Array Subset "M"(array=w424, index=w398) -> (w396:dbl[])  [unwired: 1 in]
                n215 = Array Subset "n"(array=w425, index=w398) -> (w379:dbl[])  [unwired: 1 in]
                n216 = Array Max & Min "nmax [1/min]"(array=w379) -> (max value=w422:dbl)  [unwired: 3 out]
                n217 = local write "Polynom"("Polynom") -> ()
                n218 = Bundle(w379, w400) -> (w383:cluster{dbl[], dbl[]})  [unwired: 1 in]
                n219 = Bundle(w379, w396) -> (w384:cluster{dbl[], dbl[]})  [unwired: 1 in]
                n220 = Multiply(x=w379, y=w397) -> (x*y=w393:dbl[])
                n221 = Array Size(array=w379) -> (size(s)=w376:i32)
                n222 = call <vilib>:"General Polynomial Fit.vi"("Y"=w396, "polynomial order"="Polynom", "X"=w379, "method"=T4."Biquadrat" ("Methode"), "algorithm"=3) -> ("Best Polynomial Fit"=w378:dbl[])  [unwired: 7 in, 3 out]
                n223 = Bundle(w379, "Best Polynomial Fit"=w378) -> (w385:cluster{dbl[], "Best Polynomial Fit":dbl[]})  [unwired: 1 in]
                n224 = Multiply(x=w378, y=w393) -> (x*y=w392:dbl[])
                n225 = Multiply(x=w376, y=0.8) -> (x*y=w387:dbl)
                n226 = Multiply(x=w376, y=0.1) -> (x*y=w370:dbl)
                n227 = Array Subset "MPoly ohne die ersten\nund letzten paar %"(array=w378, index=w370, length=w387) -> (w381:dbl[])
                n228 = Array Subset "n ohne die ersten \nund letzten paar %"(array=w379, index=w370, length=w387) -> ()  [unwired: 1 out]
                n229 = Divide(x=w422, y=w404) -> (x/y=w421:dbl)
                n230 = Divide(x=w392, y=w391) -> (x/y=w377:dbl[])
                n231 = Array Subset "PPoly ohne die ersten\nund letzten paar %"(array=w377, index=w370, length=w387) -> (w382:dbl[])
                n232 = Bundle(w379, w377) -> (w386:cluster{dbl[], dbl[]})  [unwired: 1 in]
                n233 = Compound Arithmetic op=MULTIPLY "vmax"(w421, w420, 0.06) -> (w412:dbl)
                n234 = Array Max & Min "Mmax"(array=w381) -> (max value=w389:dbl, max index (indices)=w372:i32)  [unwired: 2 out]
                n235 = Add(x=w370, y=w372) -> (x+y=w371:dbl)
                n236 = Multiply(x=w389, y=1.8) -> (x*y=w433:dbl)
                n237 = Index Array "n(Mmax)"(array=w379, index=w371) -> (element=w413:dbl)
                n238 = Array Max & Min "Pmax"(array=w382) -> (max value=w390:dbl, max index (indices)=w374:i32)  [unwired: 2 out]
                n239 = Build Array(w386, w385, w383, w384) -> (→"XY-Graph":cluster{dbl[], "Best Polynomial Fit":dbl[]}[])
                n240 = Add(x=w370, y=w374) -> (x+y=w373:dbl)
                n241 = local read "Luftfeuchtigkeit [%]"() -> (w416:dbl)
                n242 = local read "Lufttemperatur [°C]"() -> (w415:dbl)
                n243 = Multiply(x=w390, y=1.2) -> (x*y=w434:dbl)
                n244 = local read "Luftdruck [mbar]"() -> (w417:dbl)
                n245 = property on="XY-Graph" class="XYGraph (strikt)"("ActYScl"=1, "YScale.Maximum"=w433, "YScale.Minimum"=w401) -> ()  [unwired: 2 in, 2 out]
                n246 = property on="XY-Graph" class="XYGraph (strikt)"("ActYScl"=w401, "YScale.Maximum"=w434, "YScale.Minimum"=w401) -> ()  [unwired: 2 in, 2 out]
                n247 = Index Array "n(Pmax)"(array=w379, index=w373) -> (element=w418:dbl)
                n248 = Format Into String(format string="%.1f PS" ("Format-String"), w390) -> (resulting string=→"Pmax":string)  [unwired: 2 in, 1 out]
                n249 = Format Date/Time String(time format string (%c)="%x %H:%M ") -> (date/time string=w405:string)  [unwired: 2 in]
                n250 = Format Into String(format string="%.1f PS bei %d 1/min   |   %.1f Nm bei %d 1/min   |   vmax: %d km/h\\nDIN 70020 k =%.3f (%d \\B0C, %d %%, %d mbar)\\n%s" ("Format-String"), w390, w418, w389, w413, w412, w406, w415, w416, w417, w405) -> (resulting string=w402:string)  [unwired: 2 in, 1 out]
                "Ergebnis" <- w402
              }
            }
            n251 = flat-sequence {
              tunnel: w16 -> [w325]
              tunnel: w18 -> [w326]
              tunnel: w22 -> [w327]
              tunnel: w23 -> [w328]
              tunnel: w24 -> [w329]
              tunnel: w25 -> [w330]
              tunnel: w26 -> [w331]
              tunnel: w27 -> [w332]
              tunnel: w28 -> [w333]
              tunnel: w29 -> [w334]
              tunnel: w30 -> [w335]
              tunnel: [w335] -> w129
              tunnel: [w334] -> w128
              tunnel: [w333] -> w127
              tunnel: [w332] -> w126
              tunnel: [w331] -> w125
              tunnel: [w330] -> w124
              tunnel: [w329] -> w123
              tunnel: [w328] -> w122
              tunnel: [w327] -> w121
              tunnel: [w326] -> w120
              tunnel: [w325] -> w119
              tunnel: [w321] -> w4
              tunnel: w3 -> [w321]
              tunnel: w129 -> [w365]
              tunnel: w128 -> [w364]
              tunnel: w127 -> [w363]
              tunnel: w126 -> [w362]
              tunnel: w125 -> [w361]
              tunnel: w124 -> [w360]
              tunnel: w123 -> [w359]
              tunnel: w122 -> [w358]
              tunnel: w121 -> [w357]
              tunnel: w120 -> [w356]
              tunnel: w119 -> [w355]
              tunnel: w4 -> [w336]
              frame #0 {
                w323 = FALSE ("Start [F1]")
                w324 = 0  # Aktivieren
                n252 = local write "Start"(w323) -> ()
                n253 = property on="Speichern" class="Bool. (strikt)"("DisabledEnum"=w324) -> ()  [unwired: 2 in, 2 out]
                n254 = property on="Übersetzung ermitteln aus" class="Enum (strikt)"("DisabledEnum"=w324) -> ()  [unwired: 2 in, 2 out]
                n255 = property on="Konfiguration:" class="Bool. (strikt)"("DisabledEnum"=w324) -> ()  [unwired: 2 in, 2 out]
                n256 = property on="Ende" class="Bool. (strikt)"("DisabledEnum"=w324) -> ()  [unwired: 2 in, 2 out]
                n257 = property on="Drucken" class="Bool. (strikt)"("DisabledEnum"=w324) -> ()  [unwired: 2 in, 2 out]
                n258 = property on="Untersetzung\nermittelt" class="Bool. (strikt)"("BoolText.Text"="GO" ("Boolescher Text.Text"), "Blinking"=w323) -> ()  [unwired: 2 in, 2 out]
                n259 = local write "Untersetzung\nermittelt"(w323) -> ()
              }
              frame #1 {
                w339 = 0.0
                n260 = local read "Übersetzung ermitteln aus"() -> (w342:T2)
                n261 = local read "Rollenträgheit [kgm²]"() -> (w352:dbl)
                n262 = local read "Gleitender Mittelwert"() -> (w348:u8)
                n263 = local read "Messung Klimadaten"() -> (w338:bool)
                n264 = local read "Rollengeber [Inkr/U]"() -> (w353:u16)
                n265 = local read "Differenzenquotient"() -> (w347:u8)
                n266 = local read "Lufttemperatur [°C]"() -> (w345:dbl)
                n267 = local read "Luftfeuchtigkeit [%]"() -> (w344:dbl)
                n268 = local read "Reifenumfang [m]"() -> (w349:dbl)
                n269 = local read "n vom Gas [1/min]"() -> (w340:dbl)
                n270 = local read "Zündung [Imp/U]"() -> (w351:u8)
                n271 = local read "Luftdruck [mbar]"() -> (w343:dbl)
                n272 = local read "Getriebe [1:]"() -> (w350:dbl)
                n273 = local read "Polynom"() -> (w346:u8)
                n274 = local read "Dauer [s]"() -> (w341:dbl)
                n275 = Bundle("Fahrzeugdaten"="Fahrzeugdaten", "date/time string"=w362, "Rollengeber [Inkr/U]"=w353, "Rollenumfang [m]"=w360, "Rollenträgheit [kgm²]"=w352, "Zündung [Imp/U]"=w351, "Getriebe [1:]"=w350, "Reifenumfang [m]"=w349, "mean value"=w363, "Gleitender Mittelwert"=w348, "Differenzenquotient"=w347, "Polynom"=w346, w365, "element"=w361, "Lufttemperatur [°C]"=w345, "Luftfeuchtigkeit [%]"=w344, "Luftdruck [mbar]"=w343, w364, w359, "Best Polynomial Fit"=w358, w357, "Übersetzung ermitteln aus"=w342, "Dauer [s]"=w341, w339, w339, "n vom Gas [1/min]"=w340, w356, w355, "Messung Klimadaten"=w338, "VISA resource name out"=w336) -> (→"Datenspeicher":T6)  [unwired: 1 in]
              }
            }
          }
        }
      }
      event "Ende": Value Change {
        n276 = event-data() -> ()  [unwired: 1 in, 6 out]
      }
    }
  }
  n277 = flat-sequence {
    frame #0 {
      n278 = call <vilib>:"Application Directory.vi"() -> ("Application Directory"=w823:path)
      n279 = Build Path(base path=w823, name or relative path="Konfig.xml") -> (appended path=w821:path)
      n280 = call-poly <vilib>:"Read From XML File.vi"("XML File Path"=w821) -> ("error out"=w802:errorcluster, "XML Elements"=w825:string)  [unwired: 8 in, 1 out]
      n281 = property on="Datenspeicher" class="Cluster (strikt)"() -> ("Value"=w824:T3)  [unwired: 2 in, 2 out]
      n282 = case shown="Fehler" w802 {
        tunnel: w825 -> [w828 _]
        tunnel: w824 -> [w827 _]
        tunnel: [w826 T3 {"Fahrzeugdaten"="", "date/time string"="05.02.2017 22:14 ", "Rolle [Inkr/U]"=10, "Rollenumfang [m]"=0.613, "Rollenträgheit [kgm²]"=0.402, "Zündung [Imp/U]"=5, "Getriebe [1:]"=5.343, "Reifenumfang [m] "=1.222, "element"=2.0, "Gl. Mittelwert"=35, "Differenzenquotient"=12, "Polynom"=15, "element"=0.01639344262295082, "element"=1.0177230216140456, "Lufttemperatur [°C]"=23.3, "Luftfeuchtigkeit [%]"=43.8, "Luftdruck [mbar]"=1013.45, array[1238 elements], array[1224 elements], "Best Polynomial Fit"=array[1224 elements], array[1224 elements], "Übersetzung ermitteln aus"=0, "[s]"=5.0, "nmin [1/min]"=0.0, "nmax [1/min]"=0.0, "n vom Gas [1/min]"=5000.0, array[1238 elements], array[1238 elements], "Boolesch"=TRUE, "Serielle Schnittstelle"=""} ("Datenspeicher")] -> w803
        frame No Error {
          n283 = Unflatten From XML(xml string=w828, type=w827) -> (value=w826:T3)  [unwired: 1 in, 1 out]
        }
        frame Error {
        }
      }
      n284 = property on="Datenspeicher" class="Cluster (strikt)"("Value"=w803) -> ()  [unwired: 2 in, 2 out]
      n285 = Unbundle(w803) -> ("Fahrzeugdaten"=w820:string, "Rolle [Inkr/U]"=w819:u16, "Rollenumfang [m]"=w818:dbl, "Rollenträgheit [kgm²]"=w817:dbl, "Zündung [Imp/U]"=w816:u8, "Getriebe [1:]"=w815:dbl, "Reifenumfang [m]"=w814:dbl, "element"=w801:dbl, "Gl. Mittelwert"=w813:u8, "Differenzenquotient"=w812:u8, "Polynom"=w811:u8, "Lufttemperatur [°C]"=w810:dbl, "Luftfeuchtigkeit [%]"=w809:dbl, "Luftdruck [mbar]"=w808:dbl, "Übersetzung ermitteln aus"=w805:u8, "[s]"=w807:dbl, "n vom Gas [1/min]"=w806:dbl, "Boolesch"=w804:bool, "Serielle Schnittstelle"=w800:refnum<visa-resource-name>)  [unwired: 11 out]
      n286 = property on="Polynom" class="DigWert (strikt)"("Value"=w811) -> ()  [unwired: 2 in, 2 out]
      n287 = property on="Dauer [s]" class="DigWert (strikt)"("Value"=w807) -> ()  [unwired: 2 in, 2 out]
      n288 = property on="Fahrzeugdaten" class="Str"("Value"=w820) -> ()  [unwired: 2 in, 2 out]
      n289 = property on="Rollengeber [Inkr/U]" class="DigWert (strikt)"("Value"=w819) -> ()  [unwired: 2 in, 2 out]
      n290 = property on="Rollenumfang [m]" class="DigWert (strikt)"("Value"=w818) -> ()  [unwired: 2 in, 2 out]
      n291 = property on="Rollenträgheit [kgm²]" class="DigWert (strikt)"("Value"=w817) -> ()  [unwired: 2 in, 2 out]
      n292 = property on="Zündung [Imp/U]" class="DigWert (strikt)"("Value"=w816) -> ()  [unwired: 2 in, 2 out]
      n293 = property on="Getriebe [1:]" class="DigWert (strikt)"("Value"=w815) -> ()  [unwired: 2 in, 2 out]
      n294 = property on="Reifenumfang [m]" class="DigWert (strikt)"("Value"=w814) -> ()  [unwired: 2 in, 2 out]
      n295 = property on="nKuWe/nRolle" class="DigWert (strikt)"("Value"=w801) -> ()  [unwired: 2 in, 2 out]
      n296 = property on="Gleitender Mittelwert" class="DigWert (strikt)"("Value"=w813) -> ()  [unwired: 2 in, 2 out]
      n297 = property on="Differenzenquotient" class="DigWert (strikt)"("Value"=w812) -> ()  [unwired: 2 in, 2 out]
      n298 = property on="Lufttemperatur [°C]" class="DigWert (strikt)"("Value"=w810) -> ()  [unwired: 2 in, 2 out]
      n299 = property on="Luftfeuchtigkeit [%]" class="DigWert (strikt)"("Value"=w809) -> ()  [unwired: 2 in, 2 out]
      n300 = property on="Luftdruck [mbar]" class="DigWert (strikt)"("Value"=w808) -> ()  [unwired: 2 in, 2 out]
      n301 = property on="Übersetzung ermitteln aus" class="Enum (strikt)"("Val(Sgnl)"=w805) -> ()  [unwired: 2 in, 2 out]
      n302 = property on="n vom Gas [1/min]" class="DigWert (strikt)"("Value"=w806) -> ()  [unwired: 2 in, 2 out]
      n303 = property on="Messung Klimadaten" class="Bool. (strikt)"("Val(Sgnl)"=w804) -> ()  [unwired: 2 in, 2 out]
      n304 = property on="Serielle Schnittstelle" class="VISAName"("Value"=w800) -> ()  [unwired: 2 in, 2 out]
    }
    frame #1 {
      w836 = 2  # Deaktivieren
      w838 = 0.0  # Graphen löschen
      n305 = local read "Serielle Schnittstelle"() -> (w834:refnum<visa-resource-name>)
      n306 = property on="Füllstand Lesepuffer" class="Schieber (strikt)"("Scale.Maximum"=100) -> ()  [unwired: 2 in, 2 out]
      n307 = property on="Frontpanel-Position" class="Bereich"("Origin"=T7 {"Horizontal"=8, "Vertical"=6}) -> ()  [unwired: 2 in, 2 out]
      n308 = property on="Drucken" class="Bool. (strikt)"("DisabledEnum"=w836) -> ()  [unwired: 2 in, 2 out]
      n309 = property on="Speichern" class="Bool. (strikt)"("DisabledEnum"=w836) -> ()  [unwired: 2 in, 2 out]
      n310 = Build Array(w838) -> (w837:dbl[])
      n311 = VISA Clear(VISA resource name=w834) -> (VISA resource name out=w833:refnum<visa-resource-name>, error out=w832:errorcluster)  [unwired: 1 in]
      n312 = property on="Untersetzung-Graph" class="SVDiagr (strikt)"("History Data"=w837) -> ()  [unwired: 2 in, 2 out]
      n313 = VISA Close(VISA resource name=w833, error in (no error)=w832) -> (error out=w831:errorcluster)
      n314 = case shown="Kein Fehler" w831 {
        tunnel: [T5."Enabled" ("Deaktiviert") T5."Disabled and Grayed Out" ("Deaktiviert")] -> w830
        frame No Error {
        }
        frame Error {
        }
      }
      n315 = property on="Start" class="Bool. (strikt)"("DisabledEnum"=w830) -> ()  [unwired: 2 in, 2 out]
    }
  }
  n316 = while {
    stop <- w842 stop-if-true
    n317 = event shown="[2] \"Speichern\": Wertänderung" {
      selector: _ -> [_ _ _ _ _ _ _ _]
      dyn-events: _ -> [_ _ _ _ _ _ _ _]
      timeout: _ -> [_ _ _ _ _ _ _ _]
      tunnel: [_ _ _ TRUE _ _ _ _] -> w842
      event "Konfiguration:": Value Change {
        n318 = event-data() -> ("OldVal"=w843:bool)  [unwired: 1 in, 5 out]
        n319 = flat-sequence {
          tunnel: [w847] -> w844
          tunnel: w843 -> [w847]
          tunnel: w844 -> [w870]
          frame #0 {
            n320 = call-poly <vilib>:"Read From XML File.vi"() -> ("error out"=w845:errorcluster, "XML Elements"=w848:string)  [unwired: 9 in, 1 out]
            n321 = property on="Datenspeicher" class="Cluster (strikt)"() -> ("Value"=w846:T3)  [unwired: 2 in, 2 out]
            n322 = case shown="Fehler" w845 {
              selector: w845 -> [_ w869]
              tunnel: w848 -> [w868 _]
              tunnel: w846 -> [w867 _]
              frame No Error {
                n323 = Unflatten From XML(xml string=w868, type=w867) -> (value=w866:T3)  [unwired: 1 in, 1 out]
                n324 = Unbundle(w866) -> ("Fahrzeugdaten"=w865:string, "Rolle [Inkr/U]"=w864:u16, "Rollenumfang [m]"=w863:dbl, "Rollenträgheit [kgm²]"=w862:dbl, "Zündung [Imp/U]"=w861:u8, "Getriebe [1:]"=w860:dbl, "Reifenumfang [m]"=w859:dbl, "Gl. Mittelwert"=w858:u8, "Differenzenquotient"=w857:u8, "Polynom"=w856:u8, "Lufttemperatur [°C]"=w855:dbl, "Luftfeuchtigkeit [%]"=w854:dbl, "Luftdruck [mbar]"=w853:dbl, "Übersetzung ermitteln aus"=w850:u8, "[s]"=w852:dbl, "n vom Gas [1/min]"=w851:dbl, "Boolesch"=w849:bool)  [unwired: 13 out]
                n325 = property on="Polynom" class="DigWert (strikt)"("Value"=w856) -> ()  [unwired: 2 in, 2 out]
                n326 = property on="Dauer [s]" class="DigWert (strikt)"("Value"=w852) -> ()  [unwired: 2 in, 2 out]
                n327 = property on="Fahrzeugdaten" class="Str"("Value"=w865) -> ()  [unwired: 2 in, 2 out]
                n328 = property on="Rollengeber [Inkr/U]" class="DigWert (strikt)"("Value"=w864) -> ()  [unwired: 2 in, 2 out]
                n329 = property on="Rollenumfang [m]" class="DigWert (strikt)"("Value"=w863) -> ()  [unwired: 2 in, 2 out]
                n330 = property on="Rollenträgheit [kgm²]" class="DigWert (strikt)"("Value"=w862) -> ()  [unwired: 2 in, 2 out]
                n331 = property on="Zündung [Imp/U]" class="DigWert (strikt)"("Value"=w861) -> ()  [unwired: 2 in, 2 out]
                n332 = property on="Getriebe [1:]" class="DigWert (strikt)"("Value"=w860) -> ()  [unwired: 2 in, 2 out]
                n333 = property on="Reifenumfang [m]" class="DigWert (strikt)"("Value"=w859) -> ()  [unwired: 2 in, 2 out]
                n334 = property on="Gleitender Mittelwert" class="DigWert (strikt)"("Value"=w858) -> ()  [unwired: 2 in, 2 out]
                n335 = property on="Differenzenquotient" class="DigWert (strikt)"("Value"=w857) -> ()  [unwired: 2 in, 2 out]
                n336 = property on="Lufttemperatur [°C]" class="DigWert (strikt)"("Value"=w855) -> ()  [unwired: 2 in, 2 out]
                n337 = property on="Luftfeuchtigkeit [%]" class="DigWert (strikt)"("Value"=w854) -> ()  [unwired: 2 in, 2 out]
                n338 = property on="Luftdruck [mbar]" class="DigWert (strikt)"("Value"=w853) -> ()  [unwired: 2 in, 2 out]
                n339 = property on="Übersetzung ermitteln aus" class="Enum (strikt)"("Val(Sgnl)"=w850) -> ()  [unwired: 2 in, 2 out]
                n340 = property on="n vom Gas [1/min]" class="DigWert (strikt)"("Value"=w851) -> ()  [unwired: 2 in, 2 out]
                n341 = property on="Messung Klimadaten" class="Bool. (strikt)"("Val(Sgnl)"=w849) -> ()  [unwired: 2 in, 2 out]
              }
              frame Error {
                n342 = call <vilib>:"Clear Errors.vi"("error in (no error)"=w869) -> ()  [unwired: 5 in, 2 out]
              }
            }
          }
          frame #1 {
            n343 = property on="Konfiguration:" class="Bool. (strikt)"("Value"=w870) -> ()  [unwired: 2 in, 2 out]
          }
        }
      }
      event "Drucken": Value Change {
        n344 = event-data() -> ("OldVal"=w871:bool)  [unwired: 1 in, 5 out]
        n345 = flat-sequence {
          tunnel: [w876] -> w872
          tunnel: w871 -> [w876]
          tunnel: w872 -> [w877]
          frame #0 {
            n346 = control-ref of="Fahrzeugdaten"() -> (w874:refnum<vi>)
            n347 = control-ref of="XY-Graph"() -> (w875:refnum<vi>)
            n348 = control-ref of="Ergebnis"() -> (w873:refnum<vi>)
            n349 = call "printgraph_V0.01.vi"("reference 2"=w873, "Fahrzeugdaten"=w874, "XYGraph (Eingang)"=w875) -> ()  [unwired: 9 in]
          }
          frame #1 {
            n350 = property on="Drucken" class="Bool. (strikt)"("Value"=w877) -> ()  [unwired: 2 in, 2 out]
          }
        }
      }
      event "Speichern": Value Change {
        n351 = event-data() -> ("OldVal"=w879:bool)  [unwired: 1 in, 5 out]
        n352 = local write "Speichern"(w879) -> ()
        n353 = control-ref of="Datenspeicher"() -> (w878:refnum<vi>)
        n354 = call "savecluster_V0.01.vi"("Referenz"=w878) -> ()  [unwired: 2 in]
      }
      event "Ende": Value Change {
        w881 = 0.0 ("element")
        (unwired) 0.0 ("element")
        n355 = event-data() -> ("OldVal"=w911:bool)  [unwired: 1 in, 5 out]
        n356 = local write "Ende"(w911) -> ()
        n357 = local read "Datenspeicher"() -> (w882:T3)
        n358 = Unbundle By Name(w882) -> ("Rolle [Inkr/U]"=w903:u16, "Rollenumfang [m]"=w902:dbl, "Rollenträgheit [kgm²]"=w901:dbl, "Zündung [Imp/U]"=w900:u8, "Getriebe [1:]"=w899:dbl, "Reifenumfang [m]"=w898:dbl, "Gl. Mittelwert"=w897:u8, "Differenzenquotient"=w896:u8, "Polynom"=w895:u8, "Lufttemperatur [°C]"=w894:dbl, "Luftfeuchtigkeit [%]"=w893:dbl, "Luftdruck [mbar]"=w891:dbl, "Best Polynomial Fit"=w892:dbl[], "Übersetzung ermitteln aus"=w890:u8, "[s]"=w889:dbl, "nmin [1/min]"=w888:dbl, "nmax [1/min]"=w887:dbl, "n vom Gas [1/min]"=w886:dbl, "Boolesch"=w885:bool, "Serielle Schnittstelle"=w880:refnum<visa-resource-name>)  [unwired: 3 out]
        n359 = call <vilib>:"Application Directory.vi"() -> ("Application Directory"=w908:path)
        n360 = Bundle By Name(cluster=w882, "Fahrzeugdaten"="", "date/time string"="", "Rolle [Inkr/U]"=w903, "Rollenumfang [m]"=w902, "Rollenträgheit [kgm²]"=w901, "Zündung [Imp/U]"=w900, "Getriebe [1:]"=w899, "Reifenumfang [m]"=w898, "element"=0.0, "Gl. Mittelwert"=w897, "Differenzenquotient"=w896, "Polynom"=w895, "element"=w881, "element"=w881, "Lufttemperatur [°C]"=w894, "Luftfeuchtigkeit [%]"=w893, "Luftdruck [mbar]"=w891, "Best Polynomial Fit"=w892, "Übersetzung ermitteln aus"=w890, "[s]"=w889, "nmin [1/min]"=w888, "nmax [1/min]"=w887, "n vom Gas [1/min]"=w886, "Boolesch"=w885, "Serielle Schnittstelle"=w880) -> (w883:T3)
        n361 = Build Path(base path=w908, name or relative path="Konfig.xml") -> (appended path=w906:path)
        n362 = Flatten To XML(anything=w883) -> (xml string=w910:string)
        n363 = call-poly <vilib>:"Write to XML File.vi"("XML Input"=w910, "XML File Path"=w906) -> ("error out"=w909:errorcluster)  [unwired: 7 in, 2 out]
        n364 = case shown="Kein Fehler" w909 {
          frame No Error {
          }
          frame Error {
          }
        }
      }
      event "Serielle Schnittstelle": Value Change {
        n365 = event-data() -> ()  [unwired: 1 in, 6 out]
        n366 = property on="Start" class="Bool. (strikt)"("DisabledEnum"=T5."Enabled" ("Deaktiviert")) -> ()  [unwired: 2 in, 2 out]
      }
      event "Messung Klimadaten": Value Change {
        n367 = event-data() -> ("NewVal"=w914:bool)  [unwired: 1 in, 5 out]
        n368 = case shown="True" w914 {
          frame True {
            w915 = T5."Disabled and Grayed Out" ("Deaktiviert")
            n369 = property on="Lufttemperatur [°C]" class="DigWert (strikt)"("DisabledEnum"=w915) -> ()  [unwired: 2 in, 2 out]
            n370 = property on="Luftdruck [mbar]" class="DigWert (strikt)"("DisabledEnum"=w915) -> ()  [unwired: 2 in, 2 out]
            n371 = property on="Luftfeuchtigkeit [%]" class="DigWert (strikt)"("DisabledEnum"=w915) -> ()  [unwired: 2 in, 2 out]
          }
          frame False {
            w916 = T5."Enabled" ("Deaktiviert")
            n372 = property on="Lufttemperatur [°C]" class="DigWert (strikt)"("DisabledEnum"=w916) -> ()  [unwired: 2 in, 2 out]
            n373 = property on="Luftdruck [mbar]" class="DigWert (strikt)"("DisabledEnum"=w916) -> ()  [unwired: 2 in, 2 out]
            n374 = property on="Luftfeuchtigkeit [%]" class="DigWert (strikt)"("DisabledEnum"=w916) -> ()  [unwired: 2 in, 2 out]
          }
        }
      }
      event "Recalc": Value Change {
        n375 = event-data() -> ("OldVal"=w919:bool)  [unwired: 1 in, 5 out]
        n376 = property on="Recalc" class="Bool. (strikt)"("Value"=w919) -> ()  [unwired: 2 in, 2 out]
        n377 = property on="Datenspeicher" class="Cluster (strikt)"() -> ("Value"=w917:T3)  [unwired: 2 in, 2 out]
        n378 = call "ReCalc_V0.16.vi"("Berechnen"=TRUE, "Datenspeicher"=w917) -> ()  [unwired: 3 in]
      }
      event "Übersetzung ermitteln aus": Value Change {
        n379 = event-data() -> ("NewVal"=w921:T2)  [unwired: 1 in, 5 out]
        n380 = case shown="\"nKuWe / nRolle\"" w921 {
          tunnel: [T5."Disabled and Grayed Out" ("Deaktiviert") T5."Disabled and Grayed Out" ("Deaktiviert") T5."Enabled" ("Deaktiviert")] -> w923
          frame "nKuWe / nRolle" {
          }
          frame "Zündsignal", Default {
          }
          frame "Getriebe & Reifen" {
          }
        }
        n381 = case shown="\"Zündsignal\", Standard" w921 {
          tunnel: [T5."Enabled" ("Deaktiviert") T5."Disabled and Grayed Out" ("Deaktiviert") T5."Disabled and Grayed Out" ("Deaktiviert")] -> w922
          frame "nKuWe / nRolle" {
          }
          frame "Zündsignal", Default {
          }
          frame "Getriebe & Reifen" {
          }
        }
        n382 = case shown="\"Zündsignal\", Standard" w921 {
          tunnel: [T5."Disabled and Grayed Out" ("Deaktiviert") T5."Enabled" ("Deaktiviert") T5."Disabled and Grayed Out" ("Deaktiviert")] -> w920
          frame "nKuWe / nRolle" {
          }
          frame "Zündsignal", Default {
          }
          frame "Getriebe & Reifen" {
          }
        }
        n383 = property on="Getriebe [1:]" class="DigWert (strikt)"("DisabledEnum"=w923) -> ()  [unwired: 2 in, 2 out]
        n384 = property on="Reifenumfang [m]" class="DigWert (strikt)"("DisabledEnum"=w923) -> ()  [unwired: 2 in, 2 out]
        n385 = property on="nKuWe/nRolle" class="DigWert (strikt)"("DisabledEnum"=w922) -> ()  [unwired: 2 in, 2 out]
        n386 = property on="Dauer [s]" class="DigWert (strikt)"("DisabledEnum"=w920) -> ()  [unwired: 2 in, 2 out]
        n387 = property on="Zündung [Imp/U]" class="DigWert (strikt)"("DisabledEnum"=w920) -> ()  [unwired: 2 in, 2 out]
      }
    }
    n388 = Quit LabVIEW(quit? (T)=w842) -> ()
  }
